vi "Remove Empty.vi"(11 "array in":string[][](array[string])) -> (3 "sorted array out":string[][](array[string]))   [LabVIEW 2020]
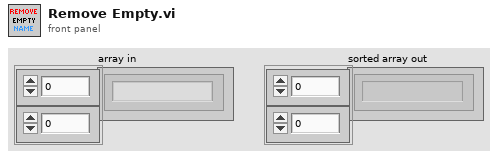
[diagram p1: front panel]
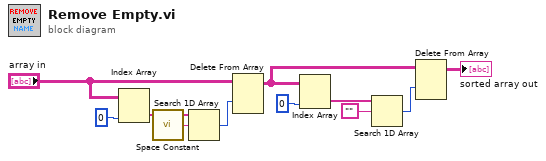
[diagram p0: block diagram]
diagram:
  n1 = Index Array(array="array in", index (col)=0 ("disabled index (col)")) -> (element=w8:string[])  [unwired: 1 in]
  n2 = call <vilib>:"Space Constant.vi"() -> ("String"=w10:string)
  n3 = Search 1D Array(1D array=w8, element=w10) -> (index of element=w11:i32)  [unwired: 1 in]
  n4 = Delete From Array(array="array in", index (row)=w11) -> (array with subset deleted=w1:string[][])  [unwired: 2 in, 1 out]
  n5 = Index Array(array=w1, index (col)=0 ("disabled index (col)")) -> (element=w5:string[])  [unwired: 1 in]
  n6 = Search 1D Array(1D array=w5, element="") -> (index of element=w6:i32)  [unwired: 1 in]
  n7 = Delete From Array(array=w1, index (row)=w6) -> (array with subset deleted=→"sorted array out":string[][])  [unwired: 2 in, 1 out]
